vi "main.vi"() -> ()   [LabVIEW 2013]
uses:
  TestMathLib/TestMathLib.lvlib
panel:
  out "Result":dbl format="%.2g"
  in  "Second number":dbl format="%.2g"
  in  "First number":dbl format="%.2g"
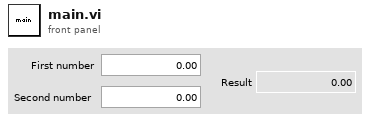
[diagram p1: front panel]
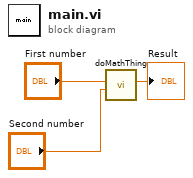
[diagram p0: block diagram]
diagram:
  n1 = call "doMathThing.vi"("Second number"="Second number", "First number"="First number") -> ("Result"=→"Result":dbl)  [unwired: 9 in]
